vi "BRig_RT_panel_ExpStruct_v1,13.vi"(7 "input_setValues":bool, 11 "input_dataExp":u16[](array[numeric])) -> (3 "output_dataExp":u16[](array[numeric]))   [LabVIEW 2014]
panel:
  in  "DAB_flipLR_nTrial":u16=100 caption="Reward Time [ms]" min=1 max=1000 step=1
  in  "I_L_nTrig_PerState":bool
  in  "I_Cue2":bool
  in  "T_Cue2_LED_max":u16=1000 caption="Max" min=5 max=5000 step=5
  in  "T_Cue2_LED_min":u16=1000 caption="Min" min=5 max=5000 step=5
  in  "T_Cue2_LED_step":u16=1000 caption="Penalty" min=1 max=10000 step=1
  in  "T_Cue2_Audio_max":u16=1000 caption="Max" min=5 max=5000 step=5
  in  "T_Cue2_Audio_min":u16=1000 caption="Min" min=5 max=5000 step=5
  in  "T_Cue2_Audio_step":u16=1000 caption="Penalty" min=1 max=10000 step=1
  in  "T_ENL2_step":u16=100 caption="Penalty" min=10 max=10000 step=10
  in  "T_ENL2_max":u16=1000 caption="Max" min=250 max=10000 step=250
  in  "T_ENL2_min":u16=1000 caption="Min" min=250 max=10000 step=250
  in  "ClosedLoop_LaserHold_l2":bool
  in  "ClosedLoop_LaserHold_l1":bool
  in  "FreeReward_Count2":u16
  in  "FreeReward_Count1":u16
  in  "FreeReward_Switch":bool
  in  "T_CuePenalty":u16=1000 caption="Penalty" min=1 max=10000 step=1
  in  "T_ENLPenalty":u16=100 caption="Penalty" min=10 max=10000 step=10
  in  "LaserSwitch_Probability_L1":u16
  in  "LaserSwitch":u16(slide) max=3 step=1 scale=0.0..3.0
  in  "I_allReward":bool caption="NonSpecific\nLick Direction"
  in  "Tcycle_Reward_max_R":u16=1000 caption="Max" min=5 max=5000 step=5
  in  "Tcycle_Reward_min_R":u16=1000 caption="Min" min=5 max=5000 step=5
  in  "Tcycle_Reward_step_R":u16=1000 caption="Penalty" min=1 max=10000 step=1
  in  "Tcycle_Reward_max_L":u16=1000 caption="Max" min=5 max=5000 step=5
  in  "Tcycle_Reward_min_L":u16=1000 caption="Min" min=5 max=5000 step=5
  in  "Tcycle_Reward_step_L":u16=1000 caption="Penalty" min=1 max=10000 step=1
  in  "T_Cue_LED_max":u16=1000 caption="Max" min=5 max=5000 step=5
  in  "T_Cue_LED_min":u16=1000 caption="Min" min=5 max=5000 step=5
  in  "T_Cue_LED_step":u16=1000 caption="Penalty" min=1 max=10000 step=1
  in  "SolenoidProbability_L":u16=100 caption="Reward Time [ms]" min=1 max=1000 step=1
  in  "SolenoidProbability_R":u16=100 caption="Reward Time [ms]" min=1 max=1000 step=1
  in  "T_Cue_Audio_max":u16=1000 caption="Max" min=5 max=5000 step=5
  in  "T_Cue_Audio_min":u16=1000 caption="Min" min=5 max=5000 step=5
  in  "BUR_max":u16 caption="Count Reward Structure  (0 = off)"
  in  "Tcycle_Timeout":u16=1000 caption="Timeout Time [ms]" min=10 max=10000 step=1
  in  "Tcycle_Wrong":u16=1000 caption="Wrong Time [ms]" min=10 max=10000 step=1
  in  "Tcycle_Selection":u16=1000 caption="Answer Time [ms]" min=1 max=10000 step=1
  in  "Tcycle_RewardPost":u16=1000 caption="Consumption Time [ms]" min=250 max=10000 step=250
  in  "TpB_Max_R":u16=4 caption="Max TrialsPerBlock" min=1 max=12 step=1
  in  "TpB_Min_R":u16=4 caption="Min TrialsPerBlock" min=1 max=12 step=1
  in  "TpB_Max_L":u16=4 caption="Max TrialsPerBlock" min=1 max=12 step=1
  in  "TpB_Min_L":u16=4 caption="Min TrialsPerBlock" min=1 max=12 step=1
  in  "BUR_min":u16 caption="Count Reward Structure\n(0 = off)"
  in  "TrialUntilReward":bool caption="Ignore Wrong\nSelection"
  in  "T_Cue_Audio_step":u16=1000 caption="Penalty" min=1 max=10000 step=1
  in  "T_ENL_step":u16=100 caption="Penalty" min=10 max=10000 step=10
  in  "T_ENL_max":u16=1000 caption="Max" min=250 max=10000 step=250
  in  "T_ENL_min":u16=1000 caption="Min" min=250 max=10000 step=250
  # "Experiment Task Structure"
  # "Min            Max               Step        Penalty"
  # "(Laser1 or Laser2)\nLaser1 probability"
  # "Enforced\nNonLick"
  # "Cue Audio"
  # "(ClosedLoop Structure)"
  # "Hold Laser1"
  # "Hold Laser2"
  # "Cue LED"
  # "Allow Multiple Laser\nTriggers During\nENL and Cue?"
  # "Min            Max               Step"
  # "ENL 2"
  # "Cue 2 Audio"
  # "Dual Armed Bandit"
  # "Cue 2 LED"
  # "Flip Directionality\nAfter X trials"
  # "Selection"
  # "Reward - Dispense Water"
  # "Min            Max            StepSize"
  # "Ignore Wrong\nSelections?"
  # "Left"
  # "Right"
  # "Dispense Water Probability"
  # "%"
  # "Left"
  # "Min"
  # "Max"
  # "Right"
  # "%"
  # "Trial Per Block Structure \n               Left                        Right"
  # "Reward - Consumption"
  # "Min"
  # "Penalty - Wrong Choice"
  # "Max"
  # "Penalty - Choice Timeout"
  # "# consecutive ReBiasing trials"
  # "Give Reward\nIf Too Many Errors"
  # "# consecutive NonForcedError trials"
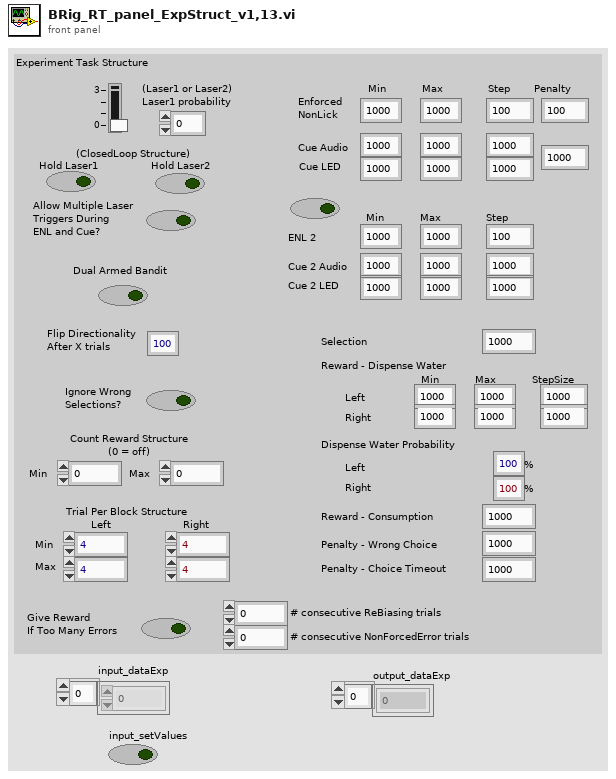
[diagram p1: front panel]
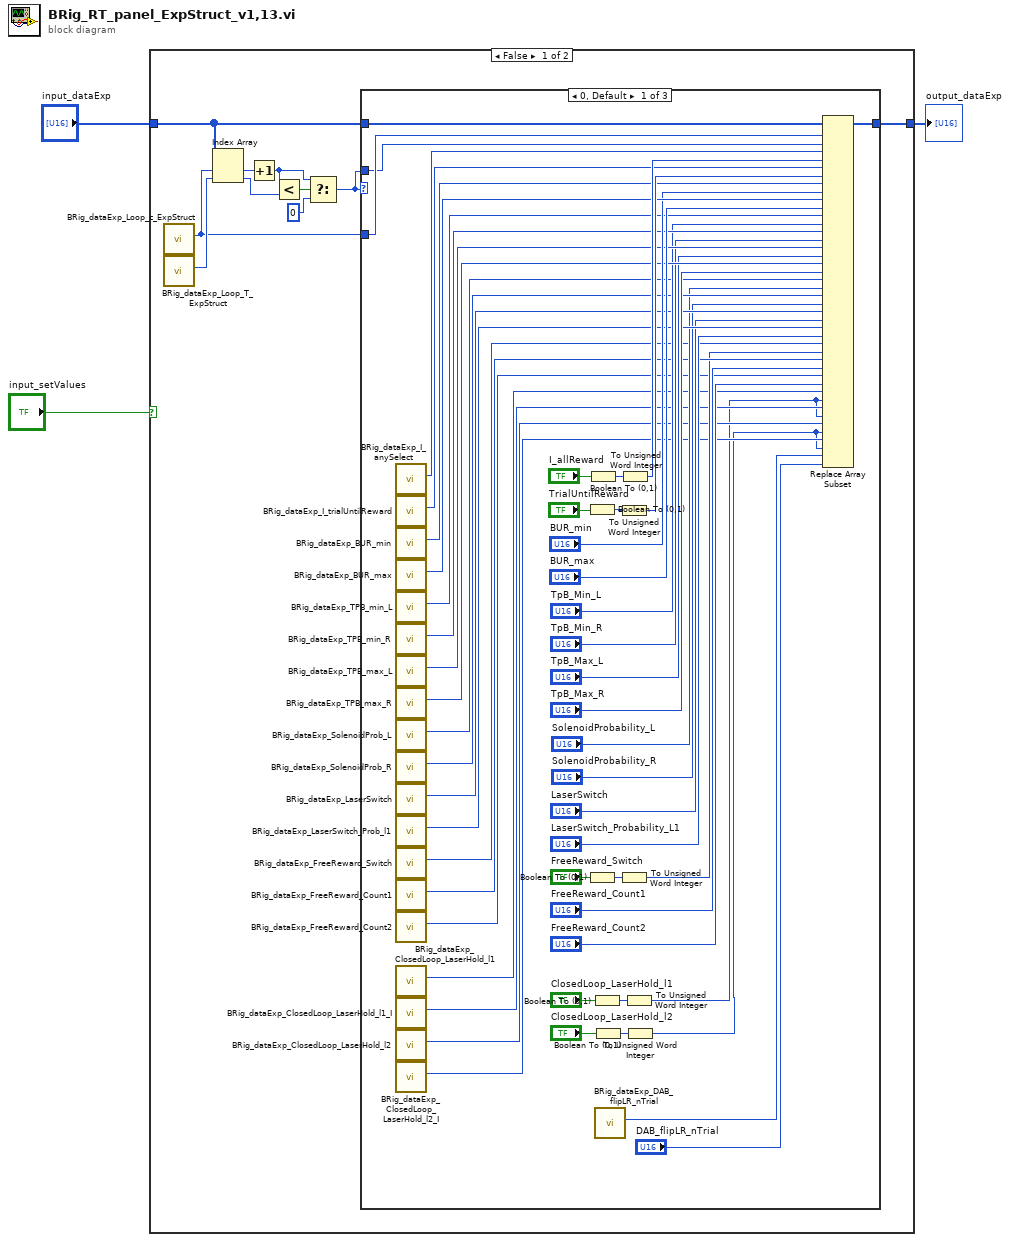
[diagram p0: block diagram]
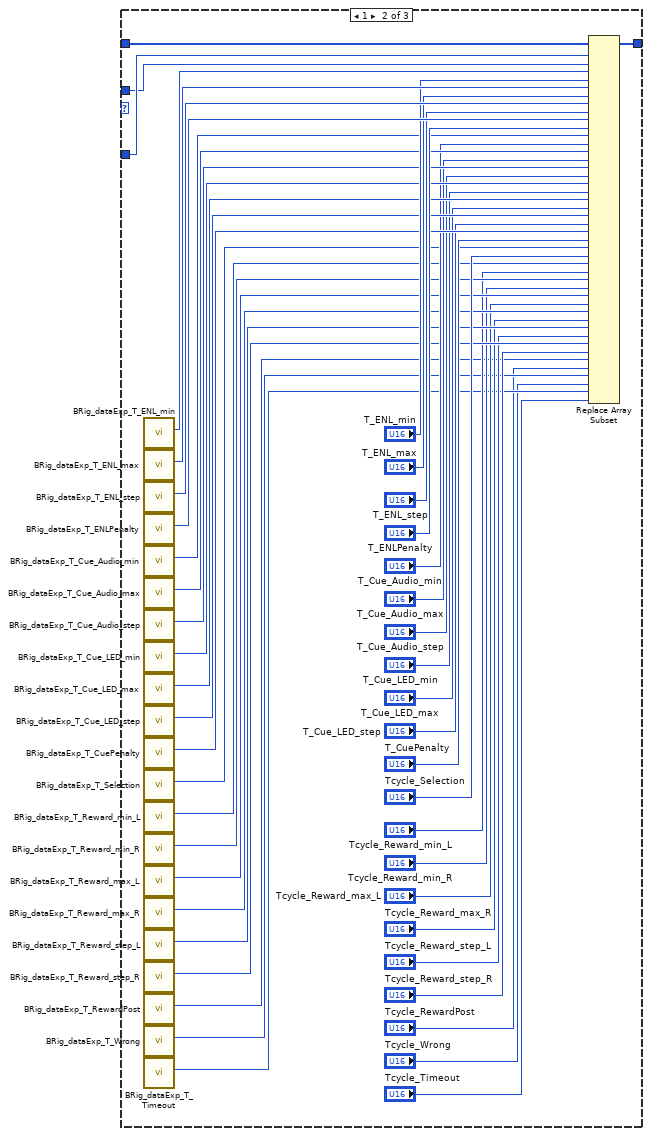
[diagram p2: hidden frame]
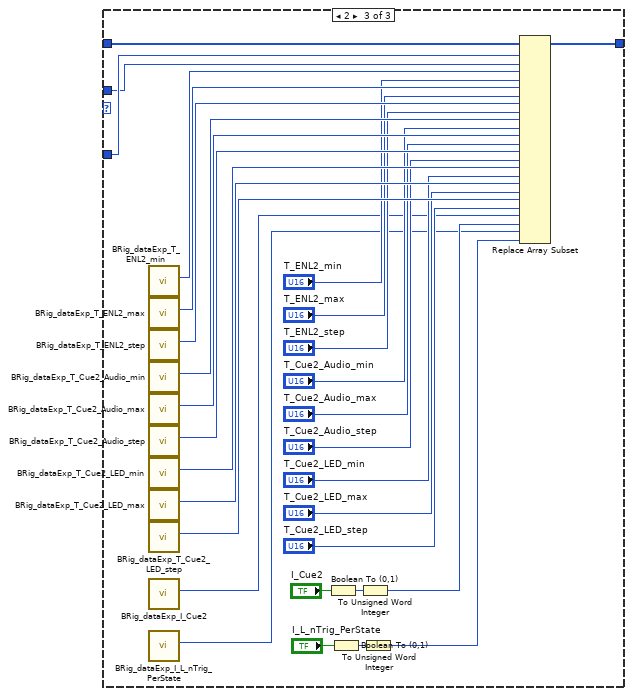
[diagram p3: hidden frame]
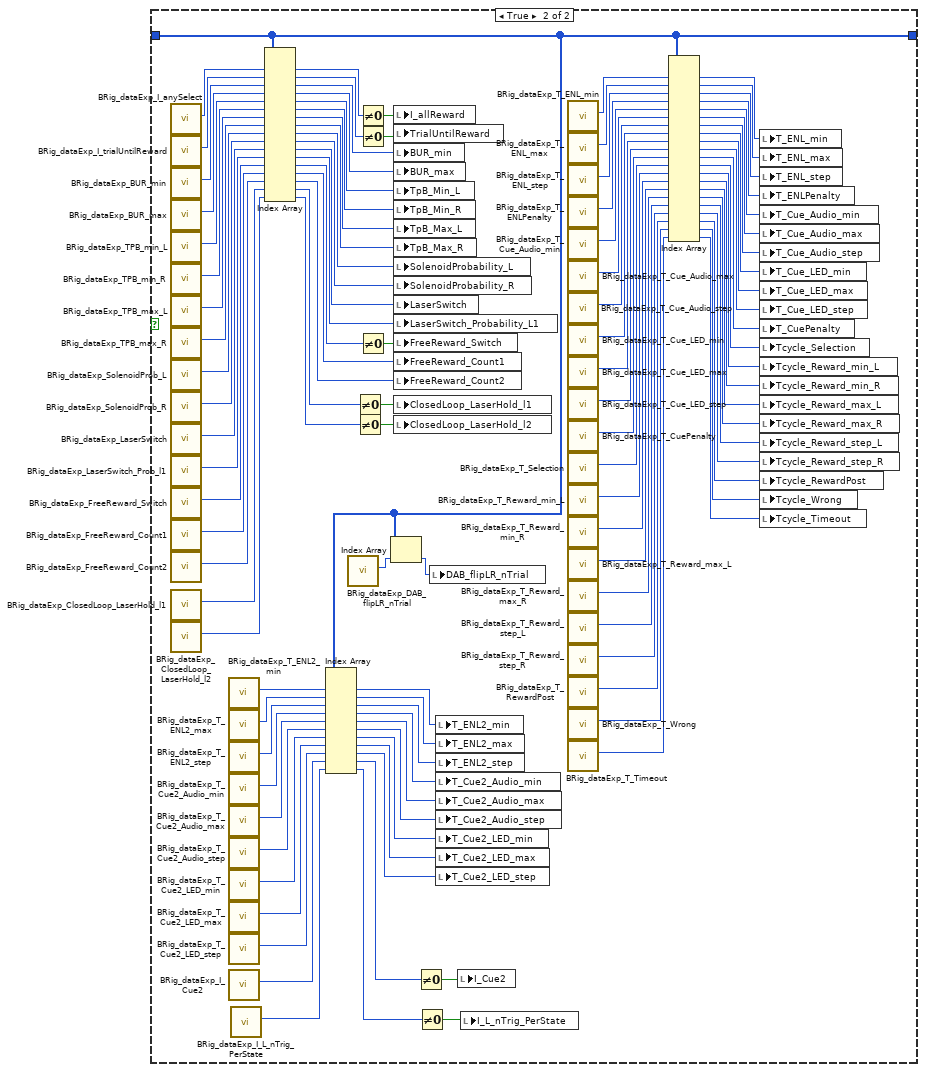
[diagram p4: hidden frame]
diagram:
  n1 = case shown="False" "input_setValues" {
    tunnel: [w13 w144] -> w3
    tunnel: "input_dataExp" -> [w12 w144]
    frame False {
      n2 = call "BRig_dataExp_Loop_c_ExpStruct.vi"() -> ("output_Loop_c_ExpStruct"=w6:i32)  [unwired: 11 in]
      n3 = call "BRig_dataExp_Loop_T_ExpStruct.vi"() -> ("output_Loop_T_ExpStruct"=w11:i32)  [unwired: 11 in]
      n4 = Index Array(array=w12, index #1=w6, index #2=w11) -> (element #1=w10:u16, element #2=w9:u16)
      n5 = Increment(x=w10) -> (x+1=w5:u16)
      n6 = Less?(x=w5, y=w9) -> (x < y?=w8:bool)
      n7 = Select(t=w5, s=w8, f=u16 0) -> (s? t:f=w4:u16)
      n8 = case shown="0, Default" w4 {
        tunnel: w12 -> [w65 w111 w141]
        tunnel: [w64 w110 w140] -> w13
        tunnel: w6 -> [w35 w109 w139]
        tunnel: w4 -> [w34 w108 w138]
        frame 0, Default {
          n9 = call "BRig_dataExp_I_anySelect.vi"() -> ("output_I_anySelect"=w63:i32)  [unwired: 11 in]
          n10 = call "BRig_dataExp_I_trialUntilReward.vi"() -> ("output_I_trialUntilReward"=w59:i32)  [unwired: 11 in]
          n11 = call "BRig_dataExp_BUR_min.vi"() -> ("output_BUR_min"=w55:i32)  [unwired: 11 in]
          n12 = call "BRig_dataExp_BUR_max.vi"() -> ("output_BUR_max"=w54:i32)  [unwired: 11 in]
          n13 = call "BRig_dataExp_TPB_min_L.vi"() -> ("output_TPB_min_L"=w51:i32)  [unwired: 11 in]
          n14 = call "BRig_dataExp_TPB_min_R.vi"() -> ("output_TPB_min_R"=w50:i32)  [unwired: 11 in]
          n15 = call "BRig_dataExp_TPB_max_L.vi"() -> ("output_TPB_max_L"=w49:i32)  [unwired: 11 in]
          n16 = call "BRig_dataExp_TPB_max_R.vi"() -> ("output_TPB_max_R"=w48:i32)  [unwired: 11 in]
          n17 = call "BRig_dataExp_SolenoidProb_L.vi"() -> ("output_SolenoidProbability_L"=w43:i32)  [unwired: 11 in]
          n18 = call "BRig_dataExp_SolenoidProb_R.vi"() -> ("output_SolenoidProbability_R"=w42:i32)  [unwired: 11 in]
          n19 = call "BRig_dataExp_LaserSwitch.vi"() -> ("output_LaserSwitch"=w41:i32)  [unwired: 11 in]
          n20 = call "BRig_dataExp_LaserSwitch_Prob_l1.vi"() -> ("output_LaserSwitch_Probability_L1"=w40:i32)  [unwired: 11 in]
          n21 = call "BRig_dataExp_FreeReward_Switch.vi"() -> ("output_FreeReward_Switch"=w31:i32)  [unwired: 11 in]
          n22 = call "BRig_dataExp_FreeReward_Count1.vi"() -> ("output_FreeReward_Count"=w30:i32)  [unwired: 11 in]
          n23 = call "BRig_dataExp_FreeReward_Count2.vi"() -> ("output_FreeReward_Count"=w27:i32)  [unwired: 11 in]
          n24 = call "BRig_dataExp_ClosedLoop_LaserHold_l1.vi"() -> ("output_CloseLoop_LaserHold_l1"=w25:i32)  [unwired: 11 in]
          n25 = call "BRig_dataExp_ClosedLoop_LaserHold_l1_I.vi"() -> ("output_CloseLoop_LaserHold_l1_I"=w24:i32)  [unwired: 11 in]
          n26 = call "BRig_dataExp_ClosedLoop_LaserHold_l2.vi"() -> ("output_CloseLoop_LaserHold_l2"=w23:i32)  [unwired: 11 in]
          n27 = call "BRig_dataExp_ClosedLoop_LaserHold_l2_I.vi"() -> ("output_CloseLoop_LaserHold_l2_I"=w22:i32)  [unwired: 11 in]
          n28 = Boolean To (0,1)(Boolean="TrialUntilReward") -> (0, 1=w58:i16)
          n29 = Boolean To (0,1)(Boolean="FreeReward_Switch") -> (0, 1=w33:i16)
          n30 = Boolean To (0,1)(Boolean="I_allReward") -> (0, 1=w61:i16)
          n31 = Boolean To (0,1)(Boolean="ClosedLoop_LaserHold_l1") -> (0, 1=w21:i16)
          n32 = Boolean To (0,1)(Boolean="ClosedLoop_LaserHold_l2") -> (0, 1=w19:i16)
          n33 = call "BRig_dataExp_DAB_flipLR_nTrial.vi"() -> ("output_DAB_flipLR_nTrial"=w15:i32)  [unwired: 11 in]
          n34 = To Unsigned Word Integer(number=w58) -> (unsigned 16bit integer=w56:u16)
          n35 = To Unsigned Word Integer(number=w33) -> (unsigned 16bit integer=w29:u16)
          n36 = To Unsigned Word Integer(number=w61) -> (unsigned 16bit integer=w60:u16)
          n37 = To Unsigned Word Integer(number=w21) -> (unsigned 16bit integer=w17:u16)
          n38 = To Unsigned Word Integer(number=w19) -> (unsigned 16bit integer=w16:u16)
          n39 = Replace Array Subset(array=w65, new element #1=w34, index #1=w35, new element #2=w60, index #2=w63, new element #3=w56, index #3=w59, new element #4="BUR_min", index #4=w55, new element #5="BUR_max", index #5=w54, new element #6="TpB_Min_L", index #6=w51, new element #7="TpB_Min_R", index #7=w50, new element #8="TpB_Max_L", index #8=w49, new element #9="TpB_Max_R", index #9=w48, new element #10="SolenoidProbability_L", index #10=w43, new element #11="SolenoidProbability_R", index #11=w42, new element #12="LaserSwitch", index #12=w41, new element #13="LaserSwitch_Probability_L1", index #13=w40, new element #14=w29, index #14=w31, new element #15="FreeReward_Count1", index #15=w30, new element #16="FreeReward_Count2", index #16=w27, new element #17=w17, index #17=w25, new element #18=w17, index #18=w24, new element #19=w16, index #19=w23, new element #20=w16, index #20=w22, new element #21="DAB_flipLR_nTrial", index #21=w15) -> (w64:u16[])
        }
        frame 1 {
          n40 = call "BRig_dataExp_T_ENL_min.vi"() -> ("output_T_ENL_min"=w107:i32)  [unwired: 11 in]
          n41 = call "BRig_dataExp_T_ENL_max.vi"() -> ("output_T_ENL_max"=w106:i32)  [unwired: 11 in]
          n42 = call "BRig_dataExp_T_ENL_step.vi"() -> ("output_T_ENL_step"=w105:i32)  [unwired: 11 in]
          n43 = call "BRig_dataExp_T_ENLPenalty.vi"() -> ("output_ENL_penalty"=w104:i32)  [unwired: 11 in]
          n44 = call "BRig_dataExp_T_Cue_Audio_min.vi"() -> ("output_T_Cue_Audio_min"=w99:i32)  [unwired: 11 in]
          n45 = call "BRig_dataExp_T_Cue_Audio_max.vi"() -> ("output_T_Cue_Audio_max"=w98:i32)  [unwired: 11 in]
          n46 = call "BRig_dataExp_T_Cue_Audio_step.vi"() -> ("output_T_Cue_Audio_step"=w97:i32)  [unwired: 11 in]
          n47 = call "BRig_dataExp_T_Cue_LED_min.vi"() -> ("output_T_Cue_LED_min"=w96:i32)  [unwired: 11 in]
          n48 = call "BRig_dataExp_T_Cue_LED_max.vi"() -> ("output_T_Cue_LED_max"=w95:i32)  [unwired: 11 in]
          n49 = call "BRig_dataExp_T_Cue_LED_step.vi"() -> ("output_T_Cue_LED_step"=w94:i32)  [unwired: 11 in]
          n50 = call "BRig_dataExp_T_CuePenalty.vi"() -> ("output_T_CuePenalty"=w93:i32)  [unwired: 11 in]
          n51 = call "BRig_dataExp_T_Selection.vi"() -> ("output_T_Selection"=w85:i32)  [unwired: 11 in]
          n52 = call "BRig_dataExp_T_Reward_min_L.vi"() -> ("output_Tcycle_Reward_min_L"=w83:i32)  [unwired: 11 in]
          n53 = call "BRig_dataExp_T_Reward_min_R.vi"() -> ("output_T_Reward_min_R"=w82:i32)  [unwired: 11 in]
          n54 = call "BRig_dataExp_T_Reward_max_L.vi"() -> ("output_T_Reward_max_L"=w81:i32)  [unwired: 11 in]
          n55 = call "BRig_dataExp_T_Reward_max_R.vi"() -> ("output_T_Reward_max_R"=w80:i32)  [unwired: 11 in]
          n56 = call "BRig_dataExp_T_Reward_step_L.vi"() -> ("output_T_Reward_step_L"=w79:i32)  [unwired: 11 in]
          n57 = call "BRig_dataExp_T_Reward_step_R.vi"() -> ("output_T_Reward_step_R"=w78:i32)  [unwired: 11 in]
          n58 = call "BRig_dataExp_T_RewardPost.vi"() -> ("output_T_RewardPost"=w71:i32)  [unwired: 11 in]
          n59 = call "BRig_dataExp_T_Wrong.vi"() -> ("output_T_Wrong"=w70:i32)  [unwired: 11 in]
          n60 = call "BRig_dataExp_T_Timeout.vi"() -> ("output_T_Timeout"=w69:i32)  [unwired: 11 in]
          n61 = Replace Array Subset(array=w111, new element #1=w108, index #1=w109, new element #2="T_ENL_min", index #2=w107, new element #3="T_ENL_max", index #3=w106, new element #4="T_ENL_step", index #4=w105, new element #5="T_ENLPenalty", index #5=w104, new element #6="T_Cue_Audio_min", index #6=w99, new element #7="T_Cue_Audio_max", index #7=w98, new element #8="T_Cue_Audio_step", index #8=w97, new element #9="T_Cue_LED_min", index #9=w96, new element #10="T_Cue_LED_max", index #10=w95, new element #11="T_Cue_LED_step", index #11=w94, new element #12="T_CuePenalty", index #12=w93, new element #13="Tcycle_Selection", index #13=w85, new element #14="Tcycle_Reward_min_L", index #14=w83, new element #15="Tcycle_Reward_min_R", index #15=w82, new element #16="Tcycle_Reward_max_L", index #16=w81, new element #17="Tcycle_Reward_max_R", index #17=w80, new element #18="Tcycle_Reward_step_L", index #18=w79, new element #19="Tcycle_Reward_step_R", index #19=w78, new element #20="Tcycle_RewardPost", index #20=w71, new element #21="Tcycle_Wrong", index #21=w70, new element #22="Tcycle_Timeout", index #22=w69) -> (w110:u16[])
        }
        frame 2 {
          n62 = call "BRig_dataExp_T_ENL2_min.vi"() -> ("output_T_ENL2_min"=w137:i32)  [unwired: 11 in]
          n63 = call "BRig_dataExp_T_ENL2_max.vi"() -> ("output_T_ENL2_max"=w136:i32)  [unwired: 11 in]
          n64 = call "BRig_dataExp_T_ENL2_step.vi"() -> ("output_T_ENL2_step"=w135:i32)  [unwired: 11 in]
          n65 = call "BRig_dataExp_T_Cue2_Audio_min.vi"() -> ("output_T_Cue2_Audio_min"=w134:i32)  [unwired: 11 in]
          n66 = call "BRig_dataExp_T_Cue2_Audio_max.vi"() -> ("output_T_Cue2_Audio_max"=w133:i32)  [unwired: 11 in]
          n67 = call "BRig_dataExp_T_Cue2_Audio_step.vi"() -> ("output_T_Cue2_Audio_step"=w132:i32)  [unwired: 11 in]
          n68 = call "BRig_dataExp_T_Cue2_LED_min.vi"() -> ("output_T_Cue2_LED_min"=w131:i32)  [unwired: 11 in]
          n69 = call "BRig_dataExp_T_Cue2_LED_max.vi"() -> ("output_T_Cue2_LED_max"=w130:i32)  [unwired: 11 in]
          n70 = call "BRig_dataExp_T_Cue2_LED_step.vi"() -> ("output_T_Cue2_LED_step"=w129:i32)  [unwired: 11 in]
          n71 = call "BRig_dataExp_I_Cue2.vi"() -> ("output_I_Cue2"=w119:i32)  [unwired: 11 in]
          n72 = call "BRig_dataExp_I_L_nTrig_PerState.vi"() -> ("output_I_L_nTrig_PerState"=w115:i32)  [unwired: 11 in]
          n73 = Boolean To (0,1)(Boolean="I_Cue2") -> (0, 1=w117:i16)
          n74 = Boolean To (0,1)(Boolean="I_L_nTrig_PerState") -> (0, 1=w114:i16)
          n75 = To Unsigned Word Integer(number=w117) -> (unsigned 16bit integer=w116:u16)
          n76 = To Unsigned Word Integer(number=w114) -> (unsigned 16bit integer=w112:u16)
          n77 = Replace Array Subset(array=w141, new element #1=w138, index #1=w139, new element #2="T_ENL2_min", index #2=w137, new element #3="T_ENL2_max", index #3=w136, new element #4="T_ENL2_step", index #4=w135, new element #5="T_Cue2_Audio_min", index #5=w134, new element #6="T_Cue2_Audio_max", index #6=w133, new element #7="T_Cue2_Audio_step", index #7=w132, new element #8="T_Cue2_LED_min", index #8=w131, new element #9="T_Cue2_LED_max", index #9=w130, new element #10="T_Cue2_LED_step", index #10=w129, new element #11=w116, index #11=w119, new element #12=w112, index #12=w115) -> (w140:u16[])
        }
      }
    }
    frame True {
      n78 = call "BRig_dataExp_I_anySelect.vi"() -> ("output_I_anySelect"=w249:i32)  [unwired: 11 in]
      n79 = call "BRig_dataExp_I_trialUntilReward.vi"() -> ("output_I_trialUntilReward"=w248:i32)  [unwired: 11 in]
      n80 = call "BRig_dataExp_BUR_min.vi"() -> ("output_BUR_min"=w247:i32)  [unwired: 11 in]
      n81 = call "BRig_dataExp_BUR_max.vi"() -> ("output_BUR_max"=w246:i32)  [unwired: 11 in]
      n82 = call "BRig_dataExp_TPB_min_L.vi"() -> ("output_TPB_min_L"=w245:i32)  [unwired: 11 in]
      n83 = call "BRig_dataExp_TPB_min_R.vi"() -> ("output_TPB_min_R"=w244:i32)  [unwired: 11 in]
      n84 = call "BRig_dataExp_TPB_max_L.vi"() -> ("output_TPB_max_L"=w243:i32)  [unwired: 11 in]
      n85 = call "BRig_dataExp_TPB_max_R.vi"() -> ("output_TPB_max_R"=w242:i32)  [unwired: 11 in]
      n86 = call "BRig_dataExp_SolenoidProb_L.vi"() -> ("output_SolenoidProbability_L"=w241:i32)  [unwired: 11 in]
      n87 = call "BRig_dataExp_SolenoidProb_R.vi"() -> ("output_SolenoidProbability_R"=w240:i32)  [unwired: 11 in]
      n88 = call "BRig_dataExp_LaserSwitch.vi"() -> ("output_LaserSwitch"=w239:i32)  [unwired: 11 in]
      n89 = call "BRig_dataExp_LaserSwitch_Prob_l1.vi"() -> ("output_LaserSwitch_Probability_L1"=w238:i32)  [unwired: 11 in]
      n90 = call "BRig_dataExp_FreeReward_Switch.vi"() -> ("output_FreeReward_Switch"=w237:i32)  [unwired: 11 in]
      n91 = call "BRig_dataExp_FreeReward_Count1.vi"() -> ("output_FreeReward_Count"=w236:i32)  [unwired: 11 in]
      n92 = call "BRig_dataExp_FreeReward_Count2.vi"() -> ("output_FreeReward_Count"=w176:i32)  [unwired: 11 in]
      n93 = call "BRig_dataExp_ClosedLoop_LaserHold_l1.vi"() -> ("output_CloseLoop_LaserHold_l1"=w174:i32)  [unwired: 11 in]
      n94 = call "BRig_dataExp_ClosedLoop_LaserHold_l2.vi"() -> ("output_CloseLoop_LaserHold_l2"=w173:i32)  [unwired: 11 in]
      n95 = call "BRig_dataExp_T_ENL2_min.vi"() -> ("output_T_ENL2_min"=w168:i32)  [unwired: 11 in]
      n96 = call "BRig_dataExp_T_ENL2_max.vi"() -> ("output_T_ENL2_max"=w167:i32)  [unwired: 11 in]
      n97 = call "BRig_dataExp_T_ENL2_step.vi"() -> ("output_T_ENL2_step"=w166:i32)  [unwired: 11 in]
      n98 = call "BRig_dataExp_T_Cue2_Audio_min.vi"() -> ("output_T_Cue2_Audio_min"=w165:i32)  [unwired: 11 in]
      n99 = call "BRig_dataExp_T_Cue2_Audio_max.vi"() -> ("output_T_Cue2_Audio_max"=w164:i32)  [unwired: 11 in]
      n100 = call "BRig_dataExp_T_Cue2_Audio_step.vi"() -> ("output_T_Cue2_Audio_step"=w163:i32)  [unwired: 11 in]
      n101 = call "BRig_dataExp_T_Cue2_LED_min.vi"() -> ("output_T_Cue2_LED_min"=w162:i32)  [unwired: 11 in]
      n102 = call "BRig_dataExp_T_Cue2_LED_max.vi"() -> ("output_T_Cue2_LED_max"=w161:i32)  [unwired: 11 in]
      n103 = call "BRig_dataExp_T_Cue2_LED_step.vi"() -> ("output_T_Cue2_LED_step"=w160:i32)  [unwired: 11 in]
      n104 = call "BRig_dataExp_I_Cue2.vi"() -> ("output_I_Cue2"=w150:i32)  [unwired: 11 in]
      n105 = call "BRig_dataExp_I_L_nTrig_PerState.vi"() -> ("output_I_L_nTrig_PerState"=w147:i32)  [unwired: 11 in]
      n106 = Index Array(array=w144, index #1=w249, index #2=w248, index #3=w247, index #4=w246, index #5=w245, index #6=w244, index #7=w243, index #8=w242, index #9=w241, index #10=w240, index #11=w239, index #12=w238, index #13=w237, index #14=w236, index #15=w176, index #16=w174, index #17=w173) -> (element #1=w232:u16, element #2=w231:u16, element #3=w230:u16, element #4=w229:u16, element #5=w228:u16, element #6=w227:u16, element #7=w226:u16, element #8=w225:u16, element #9=w224:u16, element #10=w223:u16, element #11=w222:u16, element #12=w221:u16, element #13=w220:u16, element #14=w219:u16, element #15=w175:u16, element #16=w170:u16, element #17=w169:u16)
      n107 = Index Array(array=w144, index #1=w168, index #2=w167, index #3=w166, index #4=w165, index #5=w164, index #6=w163, index #7=w162, index #8=w161, index #9=w160, index #10=w150, index #11=w147) -> (element #1=w159:u16, element #2=w158:u16, element #3=w157:u16, element #4=w156:u16, element #5=w155:u16, element #6=w154:u16, element #7=w153:u16, element #8=w152:u16, element #9=w151:u16, element #10=w148:u16, element #11=w146:u16)
      n108 = call "BRig_dataExp_DAB_flipLR_nTrial.vi"() -> ("output_DAB_flipLR_nTrial"=w143:i32)  [unwired: 11 in]
      n109 = Not Equal To 0?(x=w170) -> (x != 0?=w172:bool)
      n110 = Not Equal To 0?(x=w169) -> (x != 0?=w171:bool)
      n111 = Not Equal To 0?(x=w232) -> (x != 0?=w235:bool)
      n112 = Not Equal To 0?(x=w231) -> (x != 0?=w234:bool)
      n113 = Not Equal To 0?(x=w220) -> (x != 0?=w233:bool)
      n114 = Index Array(array=w144, index=w143) -> (element=w142:u16)
      n115 = local write "I_allReward"(w235) -> ()
      n116 = local write "TrialUntilReward"(w234) -> ()
      n117 = local write "BUR_min"(w230) -> ()
      n118 = local write "BUR_max"(w229) -> ()
      n119 = local write "TpB_Min_L"(w228) -> ()
      n120 = local write "TpB_Min_R"(w227) -> ()
      n121 = local write "TpB_Max_L"(w226) -> ()
      n122 = local write "TpB_Max_R"(w225) -> ()
      n123 = local write "SolenoidProbability_L"(w224) -> ()
      n124 = local write "SolenoidProbability_R"(w223) -> ()
      n125 = local write "LaserSwitch"(w222) -> ()
      n126 = local write "LaserSwitch_Probability_L1"(w221) -> ()
      n127 = local write "FreeReward_Switch"(w233) -> ()
      n128 = local write "FreeReward_Count1"(w219) -> ()
      n129 = local write "FreeReward_Count2"(w175) -> ()
      n130 = local write "ClosedLoop_LaserHold_l1"(w172) -> ()
      n131 = local write "ClosedLoop_LaserHold_l2"(w171) -> ()
      n132 = Not Equal To 0?(x=w148) -> (x != 0?=w149:bool)
      n133 = Not Equal To 0?(x=w146) -> (x != 0?=w145:bool)
      n134 = local write "DAB_flipLR_nTrial"(w142) -> ()
      n135 = local write "T_ENL2_min"(w159) -> ()
      n136 = local write "T_ENL2_max"(w158) -> ()
      n137 = local write "T_ENL2_step"(w157) -> ()
      n138 = local write "T_Cue2_Audio_min"(w156) -> ()
      n139 = local write "T_Cue2_Audio_max"(w155) -> ()
      n140 = local write "T_Cue2_Audio_step"(w154) -> ()
      n141 = local write "T_Cue2_LED_min"(w153) -> ()
      n142 = local write "T_Cue2_LED_max"(w152) -> ()
      n143 = local write "T_Cue2_LED_step"(w151) -> ()
      n144 = local write "I_Cue2"(w149) -> ()
      n145 = local write "I_L_nTrig_PerState"(w145) -> ()
      n146 = call "BRig_dataExp_T_ENL_min.vi"() -> ("output_T_ENL_min"=w218:i32)  [unwired: 11 in]
      n147 = call "BRig_dataExp_T_ENL_max.vi"() -> ("output_T_ENL_max"=w217:i32)  [unwired: 11 in]
      n148 = call "BRig_dataExp_T_ENL_step.vi"() -> ("output_T_ENL_step"=w216:i32)  [unwired: 11 in]
      n149 = call "BRig_dataExp_T_ENLPenalty.vi"() -> ("output_ENL_penalty"=w215:i32)  [unwired: 11 in]
      n150 = call "BRig_dataExp_T_Cue_Audio_min.vi"() -> ("output_T_Cue_Audio_min"=w214:i32)  [unwired: 11 in]
      n151 = call "BRig_dataExp_T_Cue_Audio_max.vi"() -> ("output_T_Cue_Audio_max"=w213:i32)  [unwired: 11 in]
      n152 = call "BRig_dataExp_T_Cue_Audio_step.vi"() -> ("output_T_Cue_Audio_step"=w212:i32)  [unwired: 11 in]
      n153 = call "BRig_dataExp_T_Cue_LED_min.vi"() -> ("output_T_Cue_LED_min"=w211:i32)  [unwired: 11 in]
      n154 = call "BRig_dataExp_T_Cue_LED_max.vi"() -> ("output_T_Cue_LED_max"=w210:i32)  [unwired: 11 in]
      n155 = call "BRig_dataExp_T_Cue_LED_step.vi"() -> ("output_T_Cue_LED_step"=w209:i32)  [unwired: 11 in]
      n156 = call "BRig_dataExp_T_CuePenalty.vi"() -> ("output_T_CuePenalty"=w208:i32)  [unwired: 11 in]
      n157 = call "BRig_dataExp_T_Selection.vi"() -> ("output_T_Selection"=w207:i32)  [unwired: 11 in]
      n158 = call "BRig_dataExp_T_Reward_min_L.vi"() -> ("output_Tcycle_Reward_min_L"=w206:i32)  [unwired: 11 in]
      n159 = call "BRig_dataExp_T_Reward_min_R.vi"() -> ("output_T_Reward_min_R"=w205:i32)  [unwired: 11 in]
      n160 = call "BRig_dataExp_T_Reward_max_L.vi"() -> ("output_T_Reward_max_L"=w204:i32)  [unwired: 11 in]
      n161 = call "BRig_dataExp_T_Reward_max_R.vi"() -> ("output_T_Reward_max_R"=w203:i32)  [unwired: 11 in]
      n162 = call "BRig_dataExp_T_Reward_step_L.vi"() -> ("output_T_Reward_step_L"=w202:i32)  [unwired: 11 in]
      n163 = call "BRig_dataExp_T_Reward_step_R.vi"() -> ("output_T_Reward_step_R"=w201:i32)  [unwired: 11 in]
      n164 = call "BRig_dataExp_T_RewardPost.vi"() -> ("output_T_RewardPost"=w200:i32)  [unwired: 11 in]
      n165 = call "BRig_dataExp_T_Wrong.vi"() -> ("output_T_Wrong"=w199:i32)  [unwired: 11 in]
      n166 = call "BRig_dataExp_T_Timeout.vi"() -> ("output_T_Timeout"=w198:i32)  [unwired: 11 in]
      n167 = Index Array(array=w144, index #1=w218, index #2=w217, index #3=w216, index #4=w215, index #5=w214, index #6=w213, index #7=w212, index #8=w211, index #9=w210, index #10=w209, index #11=w208, index #12=w207, index #13=w206, index #14=w205, index #15=w204, index #16=w203, index #17=w202, index #18=w201, index #19=w200, index #20=w199, index #21=w198) -> (element #1=w197:u16, element #2=w196:u16, element #3=w195:u16, element #4=w194:u16, element #5=w193:u16, element #6=w192:u16, element #7=w191:u16, element #8=w190:u16, element #9=w189:u16, element #10=w188:u16, element #11=w187:u16, element #12=w186:u16, element #13=w185:u16, element #14=w184:u16, element #15=w183:u16, element #16=w182:u16, element #17=w181:u16, element #18=w180:u16, element #19=w179:u16, element #20=w178:u16, element #21=w177:u16)
      n168 = local write "T_ENL_min"(w197) -> ()
      n169 = local write "T_ENL_max"(w196) -> ()
      n170 = local write "T_ENL_step"(w195) -> ()
      n171 = local write "T_ENLPenalty"(w194) -> ()
      n172 = local write "T_Cue_Audio_min"(w193) -> ()
      n173 = local write "T_Cue_Audio_max"(w192) -> ()
      n174 = local write "T_Cue_Audio_step"(w191) -> ()
      n175 = local write "T_Cue_LED_min"(w190) -> ()
      n176 = local write "T_Cue_LED_max"(w189) -> ()
      n177 = local write "T_Cue_LED_step"(w188) -> ()
      n178 = local write "T_CuePenalty"(w187) -> ()
      n179 = local write "Tcycle_Selection"(w186) -> ()
      n180 = local write "Tcycle_Reward_min_L"(w185) -> ()
      n181 = local write "Tcycle_Reward_min_R"(w184) -> ()
      n182 = local write "Tcycle_Reward_max_L"(w183) -> ()
      n183 = local write "Tcycle_Reward_max_R"(w182) -> ()
      n184 = local write "Tcycle_Reward_step_L"(w181) -> ()
      n185 = local write "Tcycle_Reward_step_R"(w180) -> ()
      n186 = local write "Tcycle_RewardPost"(w179) -> ()
      n187 = local write "Tcycle_Wrong"(w178) -> ()
      n188 = local write "Tcycle_Timeout"(w177) -> ()
    }
  }
  "output_dataExp" <- w3
